vi "Enable UI.vi"(8 "error in":errorcluster, 10 "Enable?":bool=TRUE, 11 "output cluster":refnum<vi>[](array[refnum])) -> (0 "error out":errorcluster)   [LabVIEW 2021]
doc: "This VI helps to enable or disable an array of UI reference."
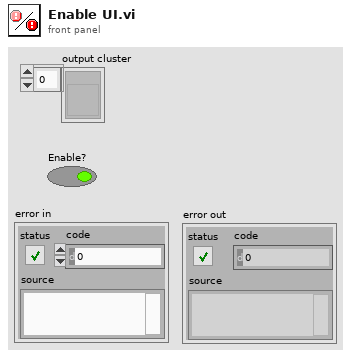
[diagram p1: front panel]
types:
  T1 = enum8{"Enabled", "Disabled", "Disabled and Grayed Out"}
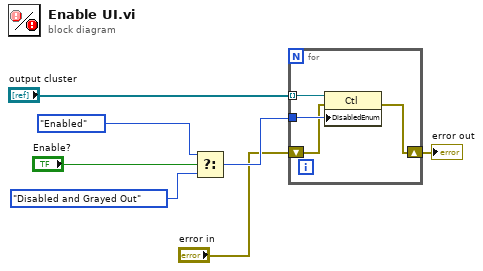
[diagram p0: block diagram]
diagram:
  n1 = Select(t=T1."Enabled" ("Disabled"), s="Enable?", f=T1."Disabled and Grayed Out") -> (s? t:f=w3:T1)
  n2 = for {
    tunnel: "output cluster" -> [w11] mode=indexing
    tunnel: w3 -> [w10]
    shift-right: [w9] -> w2
    shift-left: "error in" -> [w8]
    n3 = property class="Ctl"(reference=w11, error in=w8, "DisabledEnum"=w10) -> (error out=w9:errorcluster)  [unwired: 1 out]
  }
  "error out" <- w2
